vi "niRFSysCalReader Example.vi"() -> ()   [LabVIEW 2018, in "niRFSysCalReader.lvlib"]
doc: "This example shows how to use the NI RF System Calibration Reader to fetch data from a NI RF System Calibration XML file."
uses:
  niRFSysCalReader.lvlib
panel:
  in  "Cal Reader Settings":enum32{"Source Path", "Receiver Path"}(tab)
  in  "Source Cal Storage Path":path=path "C:/Users/Public/Documents/National Instruments/NI RF System Calibration/NI RF System Calibration Assistant/CalData/TXPath/Source_Pathloss.xml" caption="niRFSysCal Data File Path"
  in  "Source Path":string="DUT_Input_Path" caption="Path Name"
  in  "Source Frequency (Hz)":dbl=1000000000.0 caption="Frequency (Hz)" format="%#_6p"
  in  "Source Output Power (dBm)":dbl caption="Power (dBm)"
  in  "Enable Source Cal Interpolation?":bool caption="Enable Interpolation?"
  in  "Receiver Cal Storage Path":path=path "C:/Users/Public/Documents/National Instruments/NI RF System Calibration/NI RF System Calibration Assistant/CalData/RXPath/Receiver_Pathloss.xml" caption="niRFSysCal Data File Path"
  in  "Receiver Path":string="DUT_Output_Path" caption="Path Name"
  in  "Receiver Frequency (Hz)":dbl=1000000000.0 caption="Frequency (Hz)" format="%#_6p"
  in  "Receiver Reference Level (dBm)":dbl caption="Ref Level (dBm)"
  in  "Enable Receiver Cal Interpolation?":bool caption="Enable Interpolation?"
  out "Receiver  Offset (dB)":dbl
  out "Source Offset (dB)":dbl
  out "error out":errorcluster
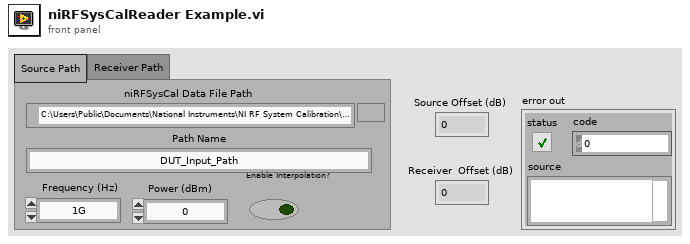
[diagram p1: front panel]
types:
  T1 = typedef "niRFSysCalReader.lvlib/niRFSysCalReader Handle.ctl" = refnum<data-value>
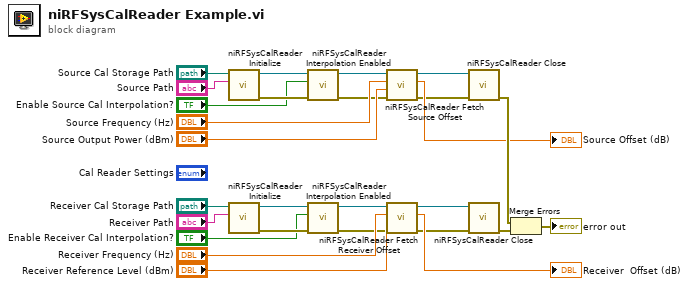
[diagram p0: block diagram]
diagram:
  n1 = call "niRFSysCalReader Initialize.vi"("Path Name"="Source Path", "niRFSysCal XML File Path"="Source Cal Storage Path") -> ("error out"=w5:errorcluster, "niRFSysCalReader Handle out"=w3:T1)  [unwired: 8 in]
  n2 = call "niRFSysCalReader Initialize.vi"("Path Name"="Receiver Path", "niRFSysCal XML File Path"="Receiver Cal Storage Path") -> ("error out"=w10:errorcluster, "niRFSysCalReader Handle out"=w8:T1)  [unwired: 8 in]
  n3 = call "niRFSysCalReader Interpolation Enabled.vi"("error in"=w5, "Enable Interpolation?"="Enable Source Cal Interpolation?", "niRFSysCalReader Handle"=w3) -> ("error out"=w4:errorcluster, "niRFSysCalReader Handle out"=w2:T1)  [unwired: 7 in]
  n4 = call "niRFSysCalReader Interpolation Enabled.vi"("error in"=w10, "Enable Interpolation?"="Enable Receiver Cal Interpolation?", "niRFSysCalReader Handle"=w8) -> ("error out"=w9:errorcluster, "niRFSysCalReader Handle out"=w7:T1)  [unwired: 7 in]
  n5 = call "niRFSysCalReader Fetch Source Offset.vi"("error in"=w4, "Desired Output Power (dBm)"="Source Output Power (dBm)", "Frequency (Hz)"="Source Frequency (Hz)", "niRFSysCalReader Handle"=w2) -> ("error out"=w20:errorcluster, "Source Offset (dB)"=→"Source Offset (dB)":dbl, "niRFSysCalReader Handle out"=w19:T1)  [unwired: 5 in]
  n6 = call "niRFSysCalReader Fetch Receiver Offset.vi"("error in"=w9, "Reference Level (dBm)"="Receiver Reference Level (dBm)", "Frequency (Hz)"="Receiver Frequency (Hz)", "niRFSysCalReader Handle"=w7) -> ("error out"=w18:errorcluster, "Receiver Offset (dB)"=→"Receiver  Offset (dB)":dbl, "niRFSysCalReader Handle out"=w17:T1)  [unwired: 5 in]
  n7 = call "niRFSysCalReader Close.vi"("error in"=w20, "niRFSysCalReader Handle"=w19) -> ("error out"=w25:errorcluster)  [unwired: 9 in]
  n8 = call "niRFSysCalReader Close.vi"("error in"=w18, "niRFSysCalReader Handle"=w17) -> ("error out"=w13:errorcluster)  [unwired: 9 in]
  n9 = Merge Errors(w25, w13) -> (→"error out":errorcluster)
